vi "Linear Mapping.vi"(7 "X":dbl, 8 "Min B":dbl, 9 "Max B":dbl, 10 "Min A":dbl, 11 "Max A":dbl) -> (2 "Y":dbl)   [LabVIEW 2018]
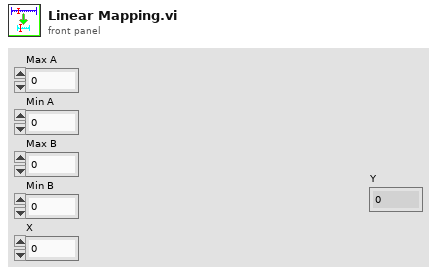
[diagram p1: front panel]
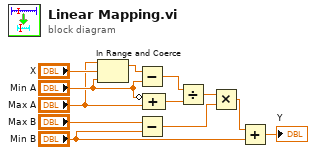
[diagram p0: block diagram]
diagram:
  n1 = In Range and Coerce(upper limit="Max A", x="X", lower limit="Min A") -> (coerced(x)=w3:dbl)  [unwired: 1 out]
  n2 = Subtract(x=w3, y="Min A") -> (x-y=w12:dbl)
  n3 = Subtract(x="Max B", y="Min B") -> (x-y=w9:dbl)
  n4 = Compound Arithmetic op=ADD(invert "Min A", "Max A") -> (w6:dbl)
  n5 = Divide(x=w12, y=w6) -> (x/y=w10:dbl)
  n6 = Multiply(x=w10, y=w9) -> (x*y=w8:dbl)
  n7 = Add(x=w8, y="Min B") -> (x+y=→"Y":dbl)
